vi "Write Node ID.vi"(8 "error in (no error)":errorcluster, 10 "Node ID":u64, 11 "DMA Channel Testing in":refnum<class "DMA Channel Testing.lvclass">) -> (0 "error out":errorcluster, 3 "DMA Channel Testing out":refnum<class "DMA Channel Testing.lvclass">)   [LabVIEW 2019, in "DMA Channel Testing.lvclass"]
uses:
  DMA Channel Testing.lvclass
  DMA Channel Testing.lvclass/DMA Channel Testing.ctl
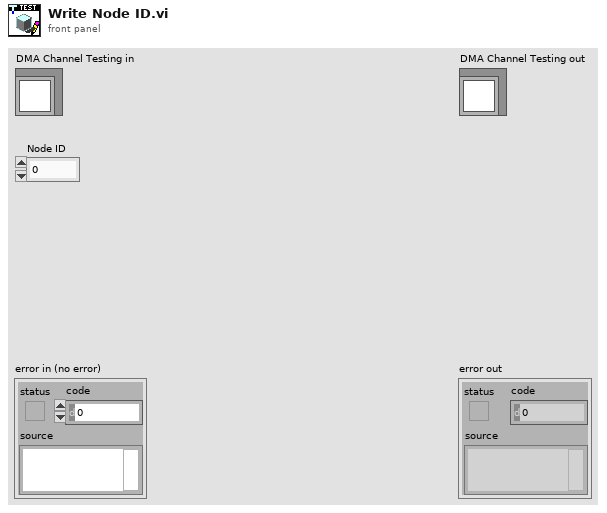
[diagram p1: front panel]
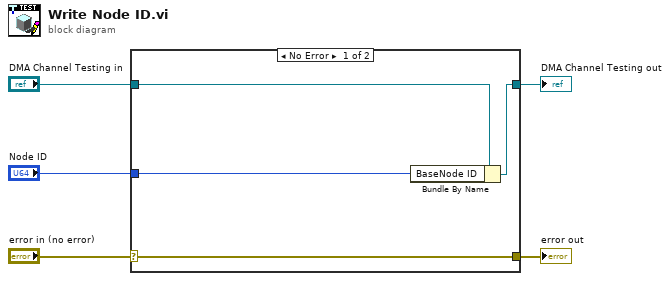
[diagram p0: block diagram]
diagram:
  n1 = case shown="No Error" "error in (no error)" {
    selector: "error in (no error)" -> [w9 w10]
    tunnel: [w9 w10] -> w4
    tunnel: [w7 w11] -> w2
    tunnel: "DMA Channel Testing in" -> [w8 w11]
    tunnel: "Node ID" -> [w6 _]
    frame No Error {
      n2 = Bundle By Name(cluster=w8, "BaseNode ID"=w6) -> (w7:refnum<class "DMA Channel Testing.lvclass">)
    }
    frame Error {
    }
  }
  "error out" <- w4
  "DMA Channel Testing out" <- w2
